vi "dare_verify_N.vi"(6 "N":T1, 7 "Answer":T1, 8 "Q":T1, 9 "R":T1, 10 "B":T1, 11 "A":T1) -> (0 "Eigenvalues":cdb[](array[numeric]), 1 "ZERO":T1, 3 "Passed":bool)   [LabVIEW 2019]
uses:
  <vilib>/Analysis/Matrix/Datatypes/RealMatrix.ctl
  <vilib>/Analysis/7linalg.llb/Eigenvalue and Vectors Output Option.ctl
  <vilib>/Analysis/7linalg.llb/Real Transpose Matrix.vi
  <vilib>/Analysis/baseanly.llb/Real A x B.vi
  <vilib>/Analysis/Matrix/Numeric/Subtract/Subtract - RM,RM.vi
  <vilib>/Analysis/Matrix/Numeric/Absolute Value/Absolute Value - RM.vi
  <vilib>/Analysis/7linalg.llb/Real Eigenvalues and Vectors.vi
  <vilib>/Analysis/Matrix/Numeric/Add/Add - RM,RM.vi
  <vilib>/Analysis/baseanly.llb/Real Inverse Matrix.vi
  <vilib>/Analysis/NI_AALPro.lvlib
  <vilib>/Analysis/NI_AALBase.lvlib
  <vilib>/Analysis/Matrix/NI_Matrix.lvlib
  <vilib>/Rock Robotics/WPI/ThirdParty/JAS_Junk/TrajLib/Trajectory_Library.lvlib
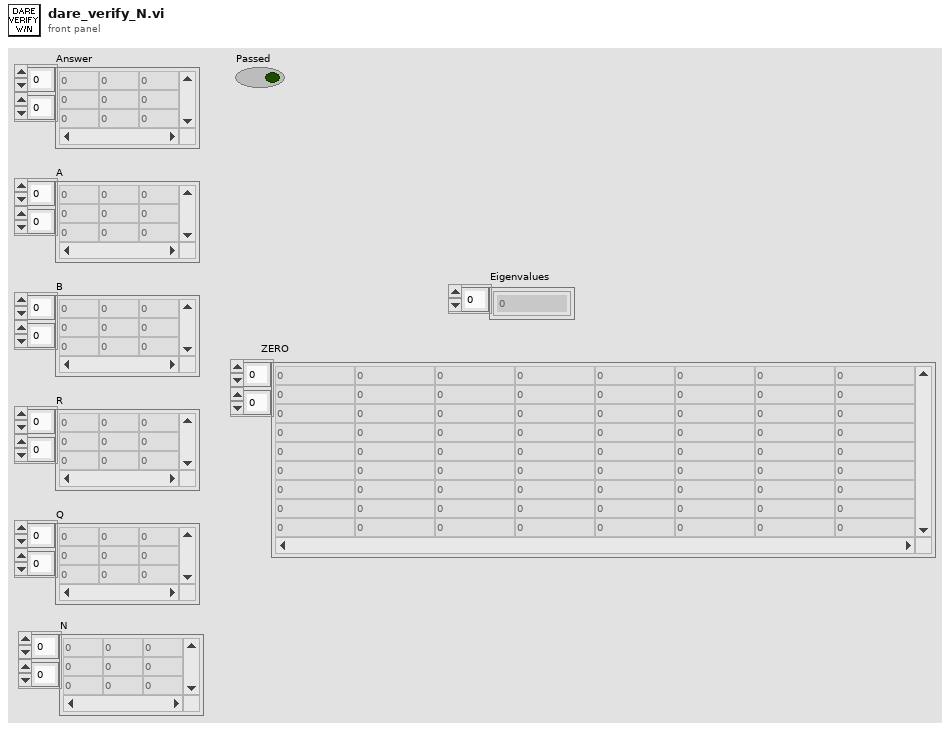
[diagram p1: front panel]
types:
  T1 = typedef "NI_Matrix.lvlib/RealMatrix.ctl" = dbl[][]
  T2 = typedef "NI_AALPro.lvlib/Eigenvalue and Vectors Output Option.ctl" = i32
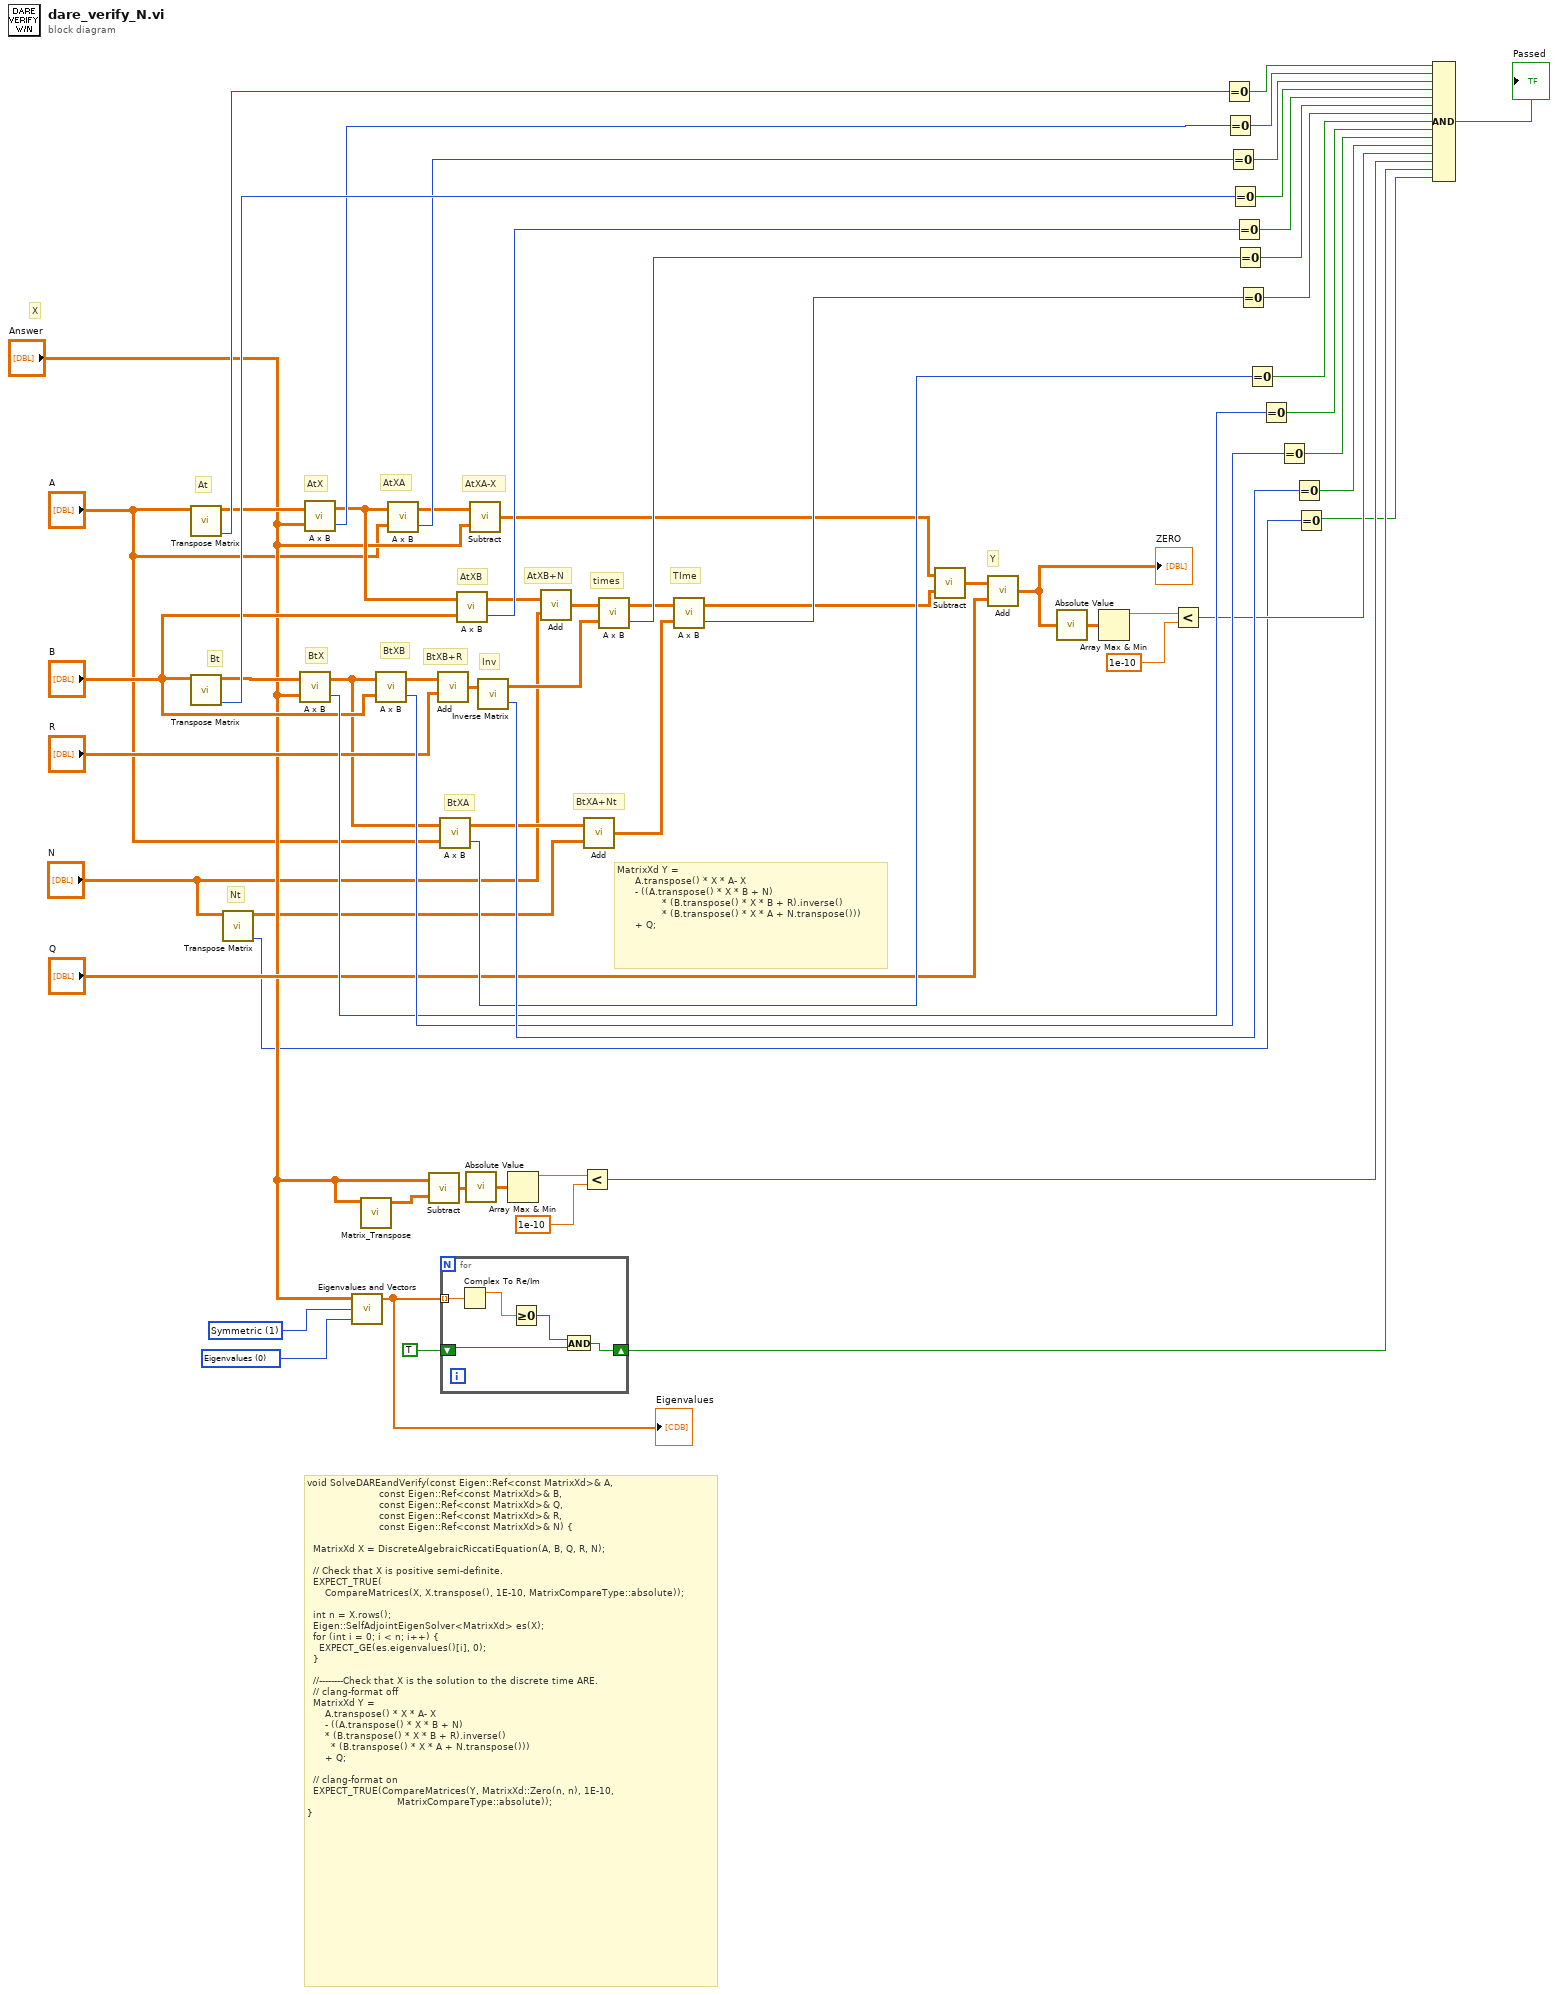
[diagram p0: block diagram]
diagram:
  w20 = T2 0 items=["Eigenvalues", "Eigenvalues & Vectors"] ("output option")
  w21 = 1 items=["General", "Symmetric"] ("matrix type")
  # "Y"
  # "Nt"
  # "TIme"
  # "BtXA+Nt"
  # "BtXA"
  # "times"
  # "AtXA-X"
  # "MatrixXd Y =\n      A.transpose() * X * A- X\n      - ((A.transpose() * X * B + N) \n               * (B.transpose() * X * B + R).inverse()\n               * (B.transpose() * X * A + N.transpose()))\n      + Q;"
  # "AtXB+N"
  # "AtXB"
  # "Inv"
  # "BtXB+R"
  # "BtX"
  # "AtXA"
  # "AtX"
  # "BtXB"
  # "X"
  # "void SolveDAREandVerify(const Eigen::Ref<const MatrixXd>& A,\n                        const Eigen::Ref<const MatrixXd>& B,\n                        const Eigen::Ref<const MatrixXd>& Q,\n                        const Eigen::Ref<const MatrixXd>& R,\n                        const Eigen::Ref<const MatrixXd>& N) {\n\n  MatrixXd X = DiscreteAlgebraicRiccatiEquation(A, B, Q, R, N);\n\n  // Check that X is positive semi-definite.\n  EXPECT_TRUE(\n      CompareMatrices(X, X.transpose(), 1E-10, MatrixCompareType::absolute));\n\n  int n = X.rows();\n  Eigen::SelfAdjointEigenSolver<MatrixXd> es(X);\n  for (int i = 0; i < n; i++) {\n    EXPECT_GE(es.eigenvalues()[i], 0);\n  }\n\n  //--------Check that X is the solution to the discrete time ARE.\n  // clang-format off\n  MatrixXd Y =\n      A.transpose() * X * A- X\n      - ((A.transpose() * X * B + N) \n      * (B.transpose() * X * B + R).inverse()\n        * (B.transpose() * X * A + N.transpose()))\n      + Q;\n\n  // clang-format on\n  EXPECT_TRUE(CompareMatrices(Y, MatrixXd::Zero(n, n), 1E-10,\n                              MatrixCompareType::absolute));\n}"
  # "Bt"
  # "At"
  n1 = call-poly <vilib>:"Transpose Matrix.vi"("Input Matrix"="A") -> ("error"=w55:i32, "Matrix Transpose"=w35:T1)  [unwired: 9 in]
  n2 = call-poly <vilib>:"Transpose Matrix.vi"("Input Matrix"="B") -> ("error"=w58:i32, "Matrix Transpose"=w32:T1)  [unwired: 9 in]
  n3 = call-poly <vilib>:"Transpose Matrix.vi"("Input Matrix"="N") -> ("error"=w13:i32, "Matrix Transpose"=w8:T1)  [unwired: 9 in]
  n4 = call-poly <vilib>:"A x B.vi"("B"="Answer", "A"=w32) -> ("error"=w62:i32, "A x B"=w9:T1)
  n5 = call-poly <vilib>:"A x B.vi"("B"="Answer", "A"=w35) -> ("error"=w56:i32, "A x B"=w34:T1)
  n6 = call-poly <vilib>:"Eigenvalues and Vectors.vi"("output option"=w20, "matrix type"=w21, "Input Matrix"="Answer") -> ("Eigenvalues"=w19:cdb[])  [unwired: 2 out]
  "Eigenvalues" <- w19
  n7 = call <vilib>:"Matrix_Transpose.vi"("input matrix"="Answer") -> ("output matrix"=w28:T1)  [unwired: 10 in]
  n8 = call-poly <vilib>:"A x B.vi"("B"="B", "A"=w9) -> ("error"=w63:i32, "A x B"=w12:T1)
  n9 = call-poly <vilib>:"A x B.vi"("B"="A", "A"=w34) -> ("error"=w57:i32, "A x B"=w29:T1)
  n10 = call-poly <vilib>:"Subtract.vi"("Real Matrix B"=w28, "Real Matrix A"="Answer") -> ("A - B"=w24:T1)
  n11 = call-poly <vilib>:"Add.vi"("Real Matrix B"="R", "Real Matrix A"=w12) -> ("A + B"=w30:T1)
  n12 = call-poly <vilib>:"A x B.vi"("B"="A", "A"=w9) -> ("error"=w61:i32, "A x B"=w6:T1)
  n13 = for {
    tunnel: w19 -> [w69] mode=indexing
    shift-right: [w65] -> w17
    shift-left: TRUE -> [w66]
    n14 = Complex To Re/Im(x + iy=w69) -> (x=w68:dbl)  [unwired: 1 out]
    n15 = Greater Or Equal To 0?(x=w68) -> (x >= 0?=w67:bool)
    n16 = And(x=w67, y=w66) -> (x .and. y?=w65:bool)
  }
  n17 = call-poly <vilib>:"A x B.vi"("B"="B", "A"=w34) -> ("error"=w59:i32, "A x B"=w15:T1)
  n18 = call-poly <vilib>:"Absolute Value.vi"("Real Matrix A"=w24) -> ("|A|"=w25:T1)
  n19 = call-poly <vilib>:"Subtract.vi"("Real Matrix B"="Answer", "Real Matrix A"=w29) -> ("A - B"=w5:T1)
  n20 = call-poly <vilib>:"Inverse Matrix.vi"("Input Matrix"=w30) -> ("error"=w64:i32, "Inverse Matrix"=w31:T1)  [unwired: 1 in]
  n21 = Array Max & Min(array=w25) -> (max value=w26:dbl)  [unwired: 3 out]
  n22 = call-poly <vilib>:"Add.vi"("Real Matrix B"="N", "Real Matrix A"=w15) -> ("A + B"=w10:T1)
  n23 = Less?(x=w26, y=1e-10) -> (x < y?=w23:bool)
  n24 = call-poly <vilib>:"Add.vi"("Real Matrix B"=w8, "Real Matrix A"=w6) -> ("A + B"=w3:T1)
  n25 = call-poly <vilib>:"A x B.vi"("B"=w31, "A"=w10) -> ("error"=w60:i32, "A x B"=w7:T1)
  n26 = call-poly <vilib>:"A x B.vi"("B"=w3, "A"=w7) -> ("error"=w16:i32, "A x B"=w4:T1)
  n27 = call-poly <vilib>:"Subtract.vi"("Real Matrix B"=w4, "Real Matrix A"=w5) -> ("A - B"=w33:T1)
  n28 = call-poly <vilib>:"Add.vi"("Real Matrix B"="Q", "Real Matrix A"=w33) -> ("A + B"=w1:T1)
  "ZERO" <- w1
  n29 = call-poly <vilib>:"Absolute Value.vi"("Real Matrix A"=w1) -> ("|A|"=w51:T1)
  n30 = Array Max & Min(array=w51) -> (max value=w52:dbl)  [unwired: 3 out]
  n31 = Less?(x=w52, y=1e-10) -> (x < y?=w54:bool)
  n32 = Equal To 0?(x=w55) -> (x = 0?=w40:bool)
  n33 = Equal To 0?(x=w56) -> (x = 0?=w41:bool)
  n34 = Equal To 0?(x=w57) -> (x = 0?=w42:bool)
  n35 = Equal To 0?(x=w58) -> (x = 0?=w43:bool)
  n36 = Equal To 0?(x=w59) -> (x = 0?=w44:bool)
  n37 = Equal To 0?(x=w60) -> (x = 0?=w45:bool)
  n38 = Equal To 0?(x=w16) -> (x = 0?=w46:bool)
  n39 = Equal To 0?(x=w61) -> (x = 0?=w47:bool)
  n40 = Equal To 0?(x=w62) -> (x = 0?=w48:bool)
  n41 = Equal To 0?(x=w63) -> (x = 0?=w49:bool)
  n42 = Equal To 0?(x=w64) -> (x = 0?=w50:bool)
  n43 = Equal To 0?(x=w13) -> (x = 0?=w14:bool)
  n44 = Compound Arithmetic op=AND(w40, w41, w42, w43, w44, w45, w46, w47, w48, w49, w50, w54, w23, w17, w14) -> (→"Passed":bool)
